vi "createHM.vi"(8 "Translation":dbl[][](array[numeric]), 11 "Theta":dbl) -> (2 "HM":dbl[][](array[numeric]))   [LabVIEW 2016]
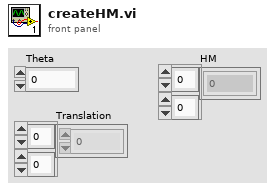
[diagram p1: front panel]
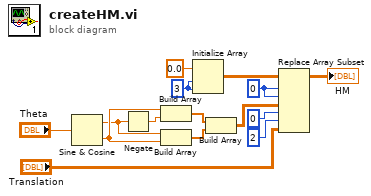
[diagram p0: block diagram]
diagram:
  w10 = 0 ("index (row)")
  w12 = 3 ("dimension size")
  n1 = Sine & Cosine(0:"Theta") -> (1:w5:dbl, 2:w9:dbl)
  n2 = Negate(x=w5) -> (-x=w6:dbl)
  n3 = Build Array(w9, w6) -> (w8:dbl[])
  n4 = Build Array(w5, w9) -> (w7:dbl[])
  n5 = Initialize Array(0.0 ("element"), w12, w12) -> (w11:dbl[][])
  n6 = Build Array(w8, w7) -> (w4:dbl[][])
  n7 = Replace Array Subset(array=w11, new element #1=w4, index (row) #1=w10, index (col) #1=w10, new element #2="Translation", index (row) #2=0 ("index (row)"), index (col) #2=2 ("disabled index (col)")) -> (→"HM":dbl[][])
